vi "check Sum.vi"(10 "Array":dbl[](array[numeric])) -> (1 "subarray":i32[](array[numeric]))   [LabVIEW 2013]
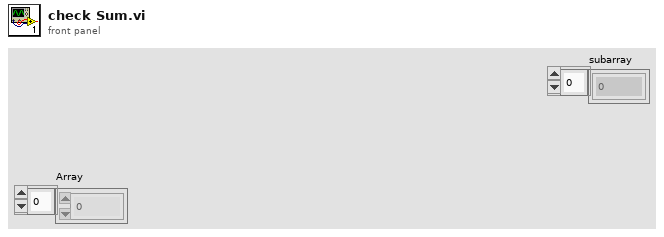
[diagram p1: front panel]
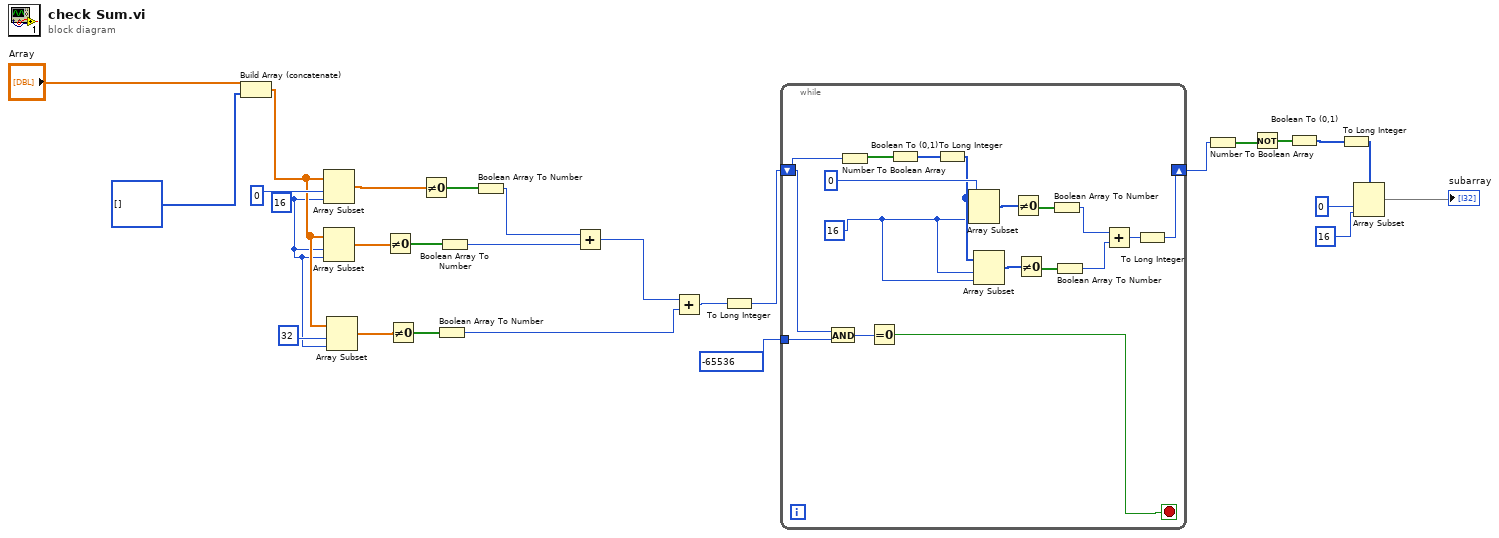
[diagram p0: block diagram]
diagram:
  w16 = 16
  n1 = Build Array (concatenate)("Array", i32[] []) -> (w18:dbl[])
  n2 = Array Subset(array=w18, index=0, length=w16) -> (w24:dbl[])
  n3 = Array Subset(array=w18, index=w16, length=w16) -> (w21:dbl[])
  n4 = Array Subset(array=w18, index=32, length=w16) -> (w15:dbl[])
  n5 = Not Equal To 0?(x=w21) -> (x != 0?=w22:bool[])
  n6 = Not Equal To 0?(x=w15) -> (x != 0?=w14:bool[])
  n7 = Not Equal To 0?(x=w24) -> (x != 0?=w23:bool[])
  n8 = Boolean Array To Number(Boolean array=w14) -> (number=w13:u32)
  n9 = Boolean Array To Number(Boolean array=w22) -> (number=w19:u32)
  n10 = Boolean Array To Number(Boolean array=w23) -> (number=w20:u32)
  n11 = Add(x=w20, y=w19) -> (x+y=w11:u32)
  n12 = Add(x=w11, y=w13) -> (x+y=w10:u32)
  n13 = To Long Integer(number=w10) -> (32bit integer=w9:i32)
  n14 = while {
    tunnel: -65536 -> [w44]
    shift-right: [w28] -> w6
    shift-left: w9 -> [w40]
    stop <- w42 stop-if-true
    w36 = 16
    n15 = And(x=w40, y=w44) -> (x .and. y?=w43:i32)
    n16 = Number To Boolean Array(number=w40) -> (Boolean array=w39:bool[])
    n17 = Equal To 0?(x=w43) -> (x = 0?=w42:bool)
    n18 = Boolean To (0,1)(Boolean=w39) -> (0, 1=w38:i16[])
    n19 = To Long Integer(number=w38) -> (32bit integer=w37:i32[])
    n20 = Array Subset(array=w37, index=0, length=w36) -> (w35:i32[])
    n21 = Array Subset(array=w37, index=w36, length=w36) -> (w32:i32[])
    n22 = Not Equal To 0?(x=w35) -> (x != 0?=w34:bool[])
    n23 = Not Equal To 0?(x=w32) -> (x != 0?=w33:bool[])
    n24 = Boolean Array To Number(Boolean array=w34) -> (number=w31:u32)
    n25 = Boolean Array To Number(Boolean array=w33) -> (number=w30:u32)
    n26 = Add(x=w31, y=w30) -> (x+y=w29:u32)
    n27 = To Long Integer(number=w29) -> (32bit integer=w28:i32)
  }
  n28 = Number To Boolean Array(number=w6) -> (Boolean array=w5:bool[])
  n29 = Not(x=w5) -> (.not. x?=w4:bool[])
  n30 = Boolean To (0,1)(Boolean=w4) -> (0, 1=w3:i16[])
  n31 = To Long Integer(number=w3) -> (32bit integer=w2:i32[])
  n32 = Array Subset(array=w2, index=0, length=16) -> (→"subarray":i32[])
